vi "Read Result Data.vi"(8 "Error In":errorcluster, 10 "Modbus ID":string, 11 "VISA resource name":refnum<visa-resource-name>) -> (0 "Error Out":errorcluster, 2 "AFV-P Result Data":T1 {"PF" format="%.3f"; "CF" format="%.2f"; "AP" format="%.1f A"; "Q" format="%.1f VAR"; "VA" format="%.1f VA"; "P" format="%.1f W"; "A" format="%.3f A"; "Voltage" format="%.1f V"; "Frequency" format="%.1f Hz"; "Time" format="%.1f s"}, 3 "VISA resource name out":refnum<visa-resource-name>)   [LabVIEW 2013]
panel:
  out "cr_dot":enum16{"CURR_XX_XX", "CURR_X_XXX"}(ring)
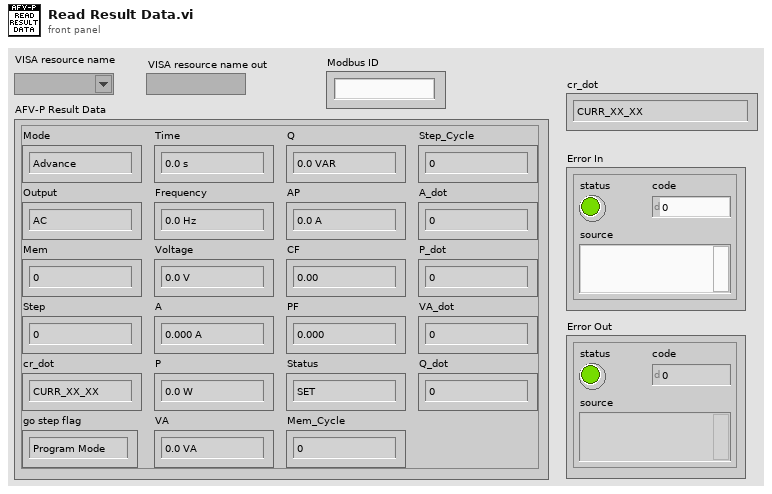
[diagram p1: front panel]
types:
  T1 = cluster{"Mode":enum16{"Advance", "Basic"}, "Output":enum16{"AC", "DC"}, "Mem":u8, "Step":u8, "go step flag":enum16{"Program Mode", "Ganaral Mode"}, "cr_dot":enum16{"CURR_XX_XX", "CURR_X_XXX"}, "Time":dbl, "Frequency":dbl, "Voltage":dbl, "A":dbl, "P":dbl, "VA":dbl, "Q":dbl, "AP":dbl, "CF":dbl, "PF":dbl, "Status":enum16{"SET", "RUNNING", "TRANSIENT", "RAMP", "DELAY", "DWELL", "PASS", "ABORT", "OCP", "A HI LIMIT", "A LO LIMIT", "VA HI LIMIT", "VA LO LIMIT", "AP HI LIMIT", "AP LO LIMIT", "P HI LIMIT", "P LO LIMIT", "PF HI LIMIT", "PF LO LIMIT", "Q HI LIMIT", "Q LO LIMIT", "CF HI LIMIT", "CF LO LIMIT", "AMP STD", "FAN FAIL", "HW OVP", "OVP", "LVP", "FA HI", "FAIL", "OPP", "FREQ-FAIL"}, "Mem_Cycle":u16, "Step_Cycle":u16, "A_dot":u8, "P_dot":u8, "VA_dot":u8, "Q_dot":u8}
  T2 = cluster{"ID":string, "Function Code":string, "Length (High)":string, "Length (Low)":string, "Start Address (High)":string, "Start Address (Middle High)":string, "Start Address (Middle Low)":string, "Start Address (Low)":string, "Data":string}
  T3 = cluster{"Length (High)":string, "Length (Low)":string, "Start Address (High)":string, "Start Address (Middle High)":string, "Start Address (Middle Low)":string, "Start Address (Low)":string}
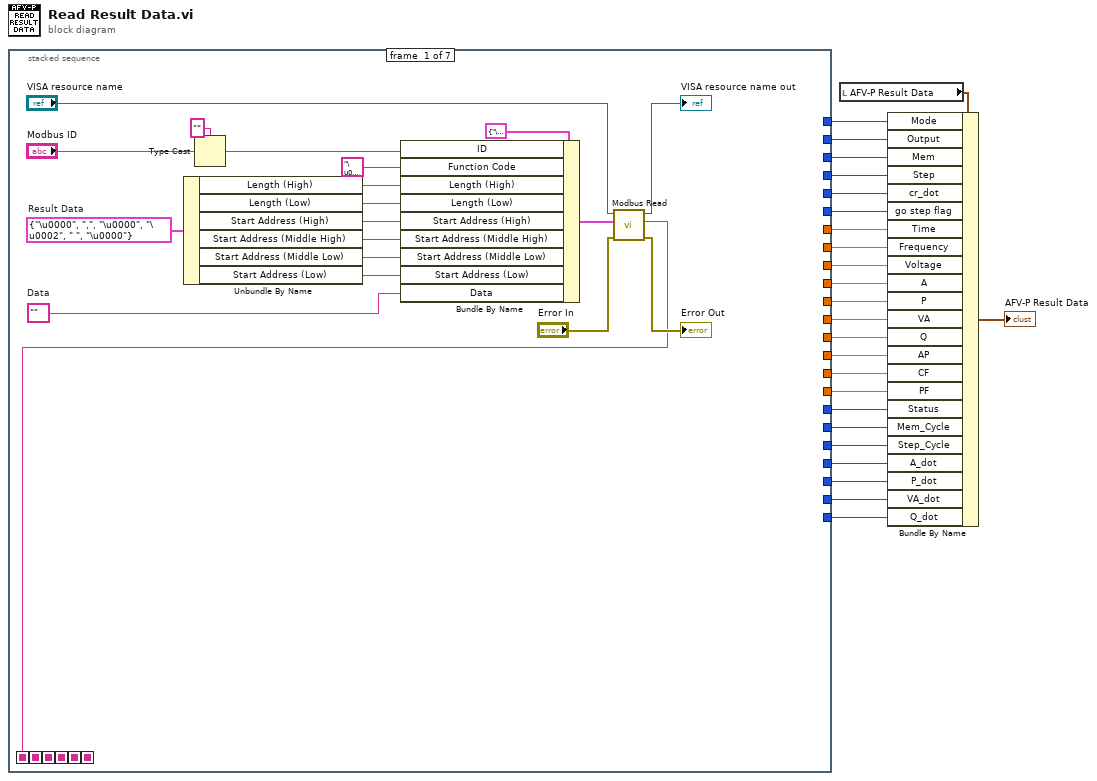
[diagram p0: block diagram]
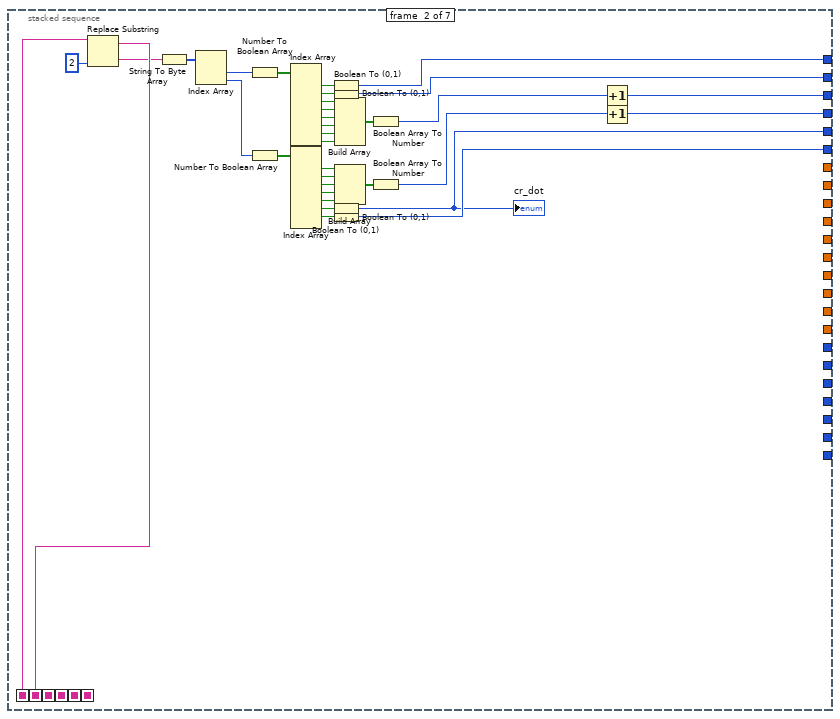
[diagram p2: hidden frame]
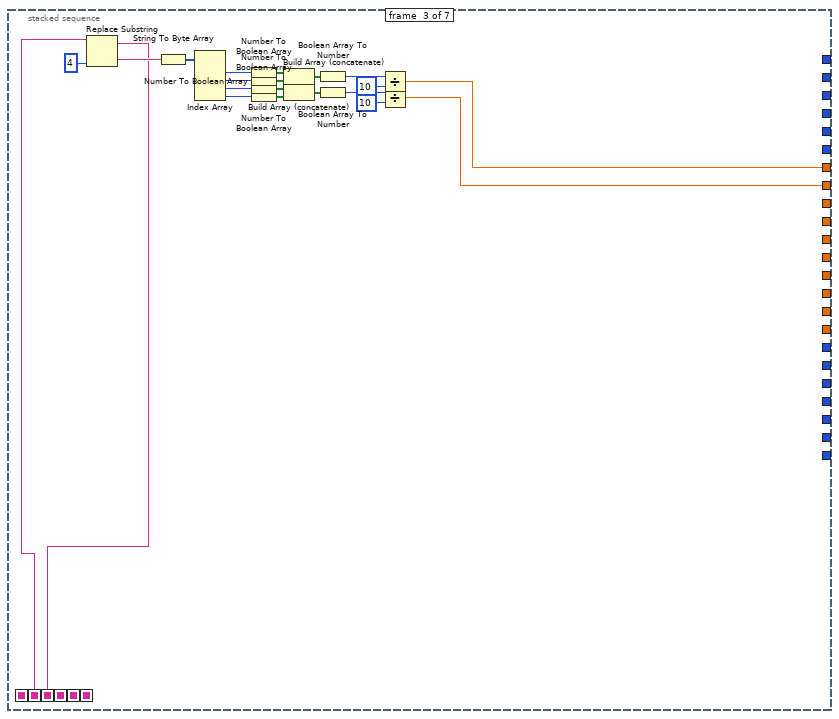
[diagram p3: hidden frame]
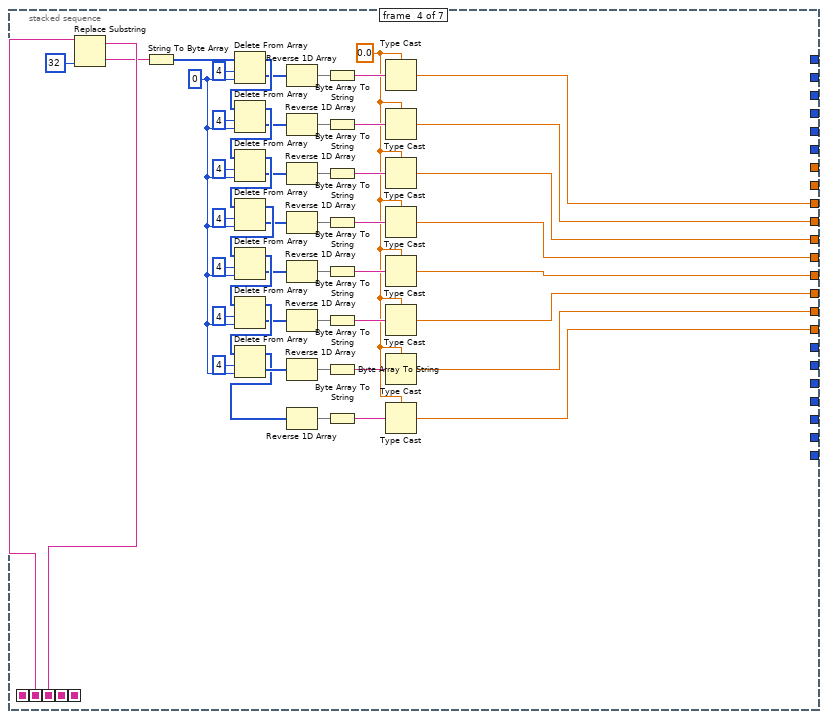
[diagram p4: hidden frame]
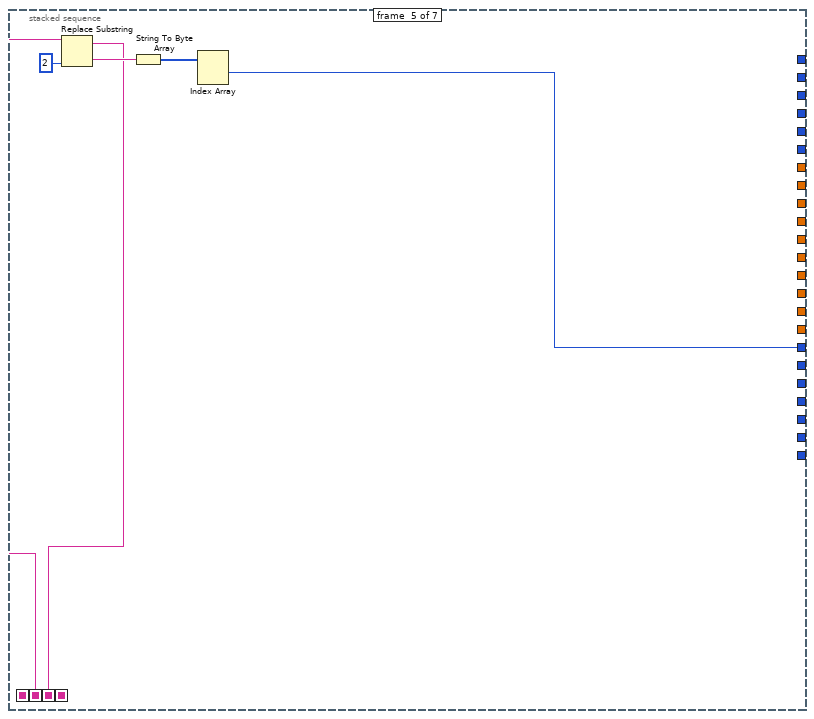
[diagram p5: hidden frame]
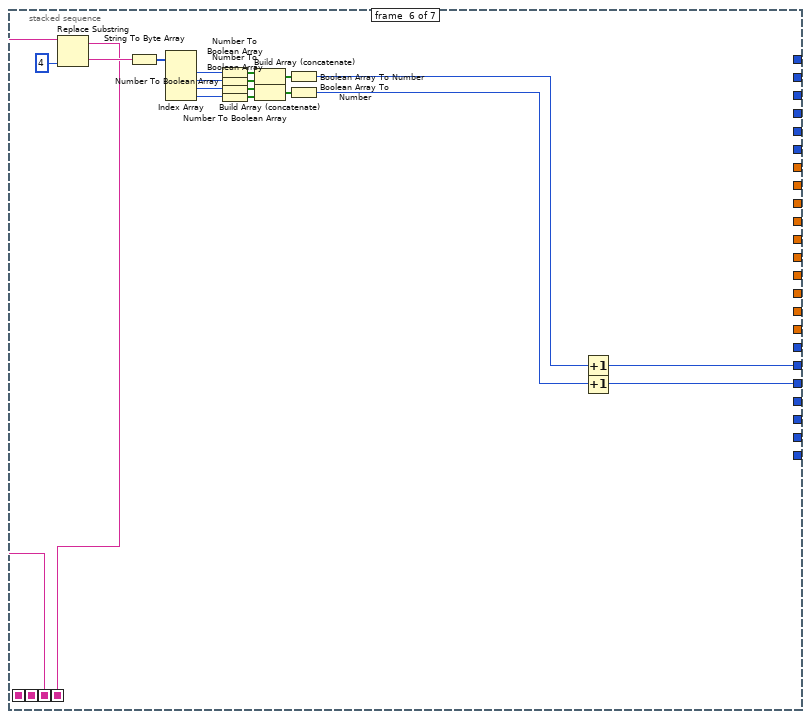
[diagram p6: hidden frame]
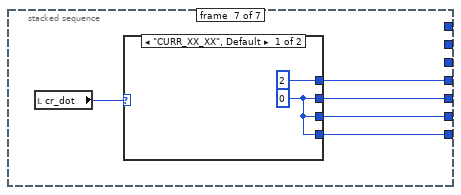
[diagram p7: hidden frame]
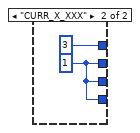
[diagram p8: hidden frame]
diagram:
  n1 = stacked-sequence {
    seq-local: [w32 _ _ _ _ _ _] -> [_ w77 _ _ _ _ _]
    seq-local: [_ w76 _ _ _ _ _] -> [_ _ w95 _ _ _ _]
    seq-local: [_ _ w96 _ _ _ _] -> [_ _ _ w149 _ _ _]
    seq-local: [_ _ _ w150 _ _ _] -> [_ _ _ _ w154 _ _]
    seq-local: [_ _ _ _ w155 _ _] -> [_ _ _ _ _ w173 _]
    seq-local: [_ _ _ _ _ w174 _] -> [_ _ _ _ _ _ _]
    tunnel: [_ w65 _ _ _ _ _] -> w25
    tunnel: [_ w49 _ _ _ _ _] -> w24
    tunnel: [_ w48 _ _ _ _ _] -> w23
    tunnel: [_ w45 _ _ _ _ _] -> w22
    tunnel: [_ _ w87 _ _ _ _] -> w21
    tunnel: [_ _ w79 _ _ _ _] -> w20
    tunnel: [_ w66 _ _ _ _ _] -> w19
    tunnel: [_ _ _ w146 _ _ _] -> w18
    tunnel: [_ _ _ w109 _ _ _] -> w17
    tunnel: [_ _ _ w108 _ _ _] -> w16
    tunnel: [_ _ _ w107 _ _ _] -> w15
    tunnel: [_ _ _ w106 _ _ _] -> w14
    tunnel: [_ _ _ w105 _ _ _] -> w13
    tunnel: [_ _ _ w104 _ _ _] -> w12
    tunnel: [_ _ _ w103 _ _ _] -> w11
    tunnel: [_ _ _ _ w152 _ _] -> w3
    tunnel: [_ _ _ _ _ w159 _] -> w10
    tunnel: [_ _ _ _ _ w158 _] -> w9
    tunnel: [_ _ _ _ _ _ w181] -> w8
    tunnel: [_ _ _ _ _ _ w180] -> w7
    tunnel: [_ _ _ _ _ _ w179] -> w6
    tunnel: [_ _ _ _ _ _ w178] -> w5
    tunnel: [_ w46 _ _ _ _ _] -> w4
    frame #0 {
      w26 = T3 {"Length (High)"="\u0000", "Length (Low)"=",", "Start Address (High)"="\u0000", "Start Address (Middle High)"="\u0002", "Start Address (Middle Low)"=" ", "Start Address (Low)"="\u0000"}  # Result Data
      w43 = ""  # Data
      n2 = Unbundle By Name(w26) -> ("Length (High)"=w42:string, "Length (Low)"=w41:string, "Start Address (High)"=w40:string, "Start Address (Middle High)"=w39:string, "Start Address (Middle Low)"=w38:string, "Start Address (Low)"=w37:string)
      n3 = Type Cast(type="" ("Binary Data (Hex) 3"), x="Modbus ID") -> (*(type *) &x=w28:string)
      n4 = Bundle By Name(cluster=T2 {"ID"="\u0000", "Function Code"="\u0000", "Length (High)"="\u0000", "Length (Low)"="\u0000", "Start Address (High)"="\u0000", "Start Address (Middle High)"="\u0000", "Start Address (Middle Low)"="\u0000", "Start Address (Low)"="\u0000", "Data"=""} ("Write Buffer"), "ID"=w28, "Function Code"="\u0003", "Length (High)"=w42, "Length (Low)"=w41, "Start Address (High)"=w40, "Start Address (Middle High)"=w39, "Start Address (Middle Low)"=w38, "Start Address (Low)"=w37, "Data"=w43) -> (w36:T2)
      n5 = call "Modbus Read.vi"("Error In"="Error In", "Write Buffer"=w36, "VISA resource name"="VISA resource name") -> ("Error Out"=→"Error Out":errorcluster, "Read Data"=w32:string, "VISA resource name out"=→"VISA resource name out":refnum<visa-resource-name>)  [unwired: 6 in]
    }
    frame #1 {
      n6 = Replace Substring(2:2 ("length (len. of substring)"), 5:w77) -> (0:w67:string, 1:w76:string)  [unwired: 2 in]
      n7 = String To Byte Array(string=w67) -> (unsigned byte array=w75:u8[])
      n8 = Index Array(array=w75) -> (element #1=w74:u8, element #2=w52:u8)  [unwired: 2 in]
      n9 = Number To Boolean Array(number=w74) -> (Boolean array=w73:bool[])
      n10 = Number To Boolean Array(number=w52) -> (Boolean array=w53:bool[])
      n11 = Index Array(array=w73) -> (element #1=w72:bool, element #2=w71:bool, element #3=w64:bool, element #4=w63:bool, element #5=w62:bool, element #6=w70:bool, element #7=w69:bool, element #8=w61:bool)  [unwired: 8 in]
      n12 = Index Array(array=w53) -> (element #1=w57:bool, element #2=w58:bool, element #3=w59:bool, element #4=w54:bool, element #5=w55:bool, element #6=w51:bool, element #7=w47:bool)  [unwired: 8 in, 1 out]
      n13 = Boolean To (0,1)(Boolean=w72) -> (0, 1=w66:i16)
      n14 = Boolean To (0,1)(Boolean=w71) -> (0, 1=w65:i16)
      n15 = Boolean To (0,1)(Boolean=w51) -> (0, 1=w45:i16)
      "cr_dot" <- w45
      n16 = Boolean To (0,1)(Boolean=w47) -> (0, 1=w46:i16)
      n17 = Build Array(w64, w63, w62, w70, w69, w61) -> (w68:bool[])
      n18 = Build Array(w57, w58, w59, w54, w55) -> (w56:bool[])
      n19 = Boolean Array To Number(Boolean array=w68) -> (number=w60:u32)
      n20 = Boolean Array To Number(Boolean array=w56) -> (number=w50:u32)
      n21 = Increment(x=w60) -> (x+1=w49:u32)
      n22 = Increment(x=w50) -> (x+1=w48:u32)
    }
    frame #2 {
      n23 = Replace Substring(2:4 ("length (len. of substring)"), 5:w95) -> (0:w97:string, 1:w96:string)  [unwired: 2 in]
      n24 = String To Byte Array(string=w97) -> (unsigned byte array=w98:u8[])
      n25 = Index Array(array=w98) -> (element #1=w91:u8, element #2=w90:u8, element #3=w81:u8, element #4=w80:u8)  [unwired: 4 in]
      n26 = Number To Boolean Array(number=w91) -> (Boolean array=w93:bool[])
      n27 = Number To Boolean Array(number=w90) -> (Boolean array=w92:bool[])
      n28 = Number To Boolean Array(number=w81) -> (Boolean array=w83:bool[])
      n29 = Number To Boolean Array(number=w80) -> (Boolean array=w84:bool[])
      n30 = Build Array (concatenate)(w93, w92) -> (w94:bool[])
      n31 = Build Array (concatenate)(w83, w84) -> (w82:bool[])
      n32 = Boolean Array To Number(Boolean array=w94) -> (number=w89:u32)
      n33 = Boolean Array To Number(Boolean array=w82) -> (number=w85:u32)
      n34 = Divide(x=w89, y=u32 10) -> (x/y=w87:dbl)
      n35 = Divide(x=w85, y=u32 10) -> (x/y=w79:dbl)
    }
    frame #3 {
      w100 = 0 ("index")
      w110 = sgl 0.0
      n36 = Replace Substring(2:32 ("length (len. of substring)"), 5:w149) -> (0:w102:string, 1:w150:string)  [unwired: 2 in]
      n37 = String To Byte Array(string=w102) -> (unsigned byte array=w101:u8[])
      n38 = Delete From Array(array=w101, length=4, index=w100) -> (deleted portion=w132:u8[], array with subset deleted=w145:u8[])
      n39 = Delete From Array(array=w145, length=4, index=w100) -> (deleted portion=w117:u8[], array with subset deleted=w139:u8[])
      n40 = Delete From Array(array=w139, length=4, index=w100) -> (deleted portion=w116:u8[], array with subset deleted=w142:u8[])
      n41 = Delete From Array(array=w142, length=4, index=w100) -> (deleted portion=w115:u8[], array with subset deleted=w133:u8[])
      n42 = Delete From Array(array=w133, length=4, index=w100) -> (deleted portion=w114:u8[], array with subset deleted=w134:u8[])
      n43 = Delete From Array(array=w134, length=4, index=w100) -> (deleted portion=w113:u8[], array with subset deleted=w138:u8[])
      n44 = Delete From Array(array=w138, length=4, index=w100) -> (deleted portion=w112:u8[], array with subset deleted=w111:u8[])
      n45 = Reverse 1D Array(array=w132) -> (reversed array=w148:u8[])
      n46 = Reverse 1D Array(array=w117) -> (reversed array=w130:u8[])
      n47 = Reverse 1D Array(array=w116) -> (reversed array=w129:u8[])
      n48 = Reverse 1D Array(array=w115) -> (reversed array=w125:u8[])
      n49 = Reverse 1D Array(array=w114) -> (reversed array=w126:u8[])
      n50 = Reverse 1D Array(array=w113) -> (reversed array=w119:u8[])
      n51 = Reverse 1D Array(array=w112) -> (reversed array=w120:u8[])
      n52 = Reverse 1D Array(array=w111) -> (reversed array=w122:u8[])
      n53 = Byte Array To String(unsigned byte array=w148) -> (string=w147:string)
      n54 = Byte Array To String(unsigned byte array=w130) -> (string=w131:string)
      n55 = Byte Array To String(unsigned byte array=w129) -> (string=w128:string)
      n56 = Byte Array To String(unsigned byte array=w125) -> (string=w124:string)
      n57 = Byte Array To String(unsigned byte array=w126) -> (string=w127:string)
      n58 = Byte Array To String(unsigned byte array=w119) -> (string=w118:string)
      n59 = Byte Array To String(unsigned byte array=w120) -> (string=w121:string)
      n60 = Byte Array To String(unsigned byte array=w122) -> (string=w123:string)
      n61 = Type Cast(type=w110, x=w147) -> (*(type *) &x=w146:sgl)
      n62 = Type Cast(type=w110, x=w131) -> (*(type *) &x=w109:sgl)
      n63 = Type Cast(type=w110, x=w128) -> (*(type *) &x=w108:sgl)
      n64 = Type Cast(type=w110, x=w124) -> (*(type *) &x=w107:sgl)
      n65 = Type Cast(type=w110, x=w127) -> (*(type *) &x=w106:sgl)
      n66 = Type Cast(type=w110, x=w118) -> (*(type *) &x=w105:sgl)
      n67 = Type Cast(type=w110, x=w121) -> (*(type *) &x=w104:sgl)
      n68 = Type Cast(type=w110, x=w123) -> (*(type *) &x=w103:sgl)
    }
    frame #4 {
      n69 = Replace Substring(2:2 ("length (len. of substring)"), 5:w154) -> (0:w156:string, 1:w155:string)  [unwired: 2 in]
      n70 = String To Byte Array(string=w156) -> (unsigned byte array=w153:u8[])
      n71 = Index Array(array=w153) -> (element #1=w152:u8)  [unwired: 2 in, 1 out]
    }
    frame #5 {
      n72 = Replace Substring(2:4 ("length (len. of substring)"), 5:w173) -> (0:w175:string, 1:w174:string)  [unwired: 2 in]
      n73 = String To Byte Array(string=w175) -> (unsigned byte array=w162:u8[])
      n74 = Index Array(array=w162) -> (element #1=w169:u8, element #2=w168:u8, element #3=w164:u8, element #4=w163:u8)  [unwired: 4 in]
      n75 = Number To Boolean Array(number=w169) -> (Boolean array=w171:bool[])
      n76 = Number To Boolean Array(number=w168) -> (Boolean array=w170:bool[])
      n77 = Number To Boolean Array(number=w164) -> (Boolean array=w166:bool[])
      n78 = Number To Boolean Array(number=w163) -> (Boolean array=w167:bool[])
      n79 = Build Array (concatenate)(w171, w170) -> (w172:bool[])
      n80 = Build Array (concatenate)(w166, w167) -> (w165:bool[])
      n81 = Boolean Array To Number(Boolean array=w172) -> (number=w161:u32)
      n82 = Boolean Array To Number(Boolean array=w165) -> (number=w160:u32)
      n83 = Increment(x=w161) -> (x+1=w159:u32)
      n84 = Increment(x=w160) -> (x+1=w158:u32)
    }
    frame #6 {
      n85 = local read "cr_dot"() -> (w177:enum16{"CURR_XX_XX", "CURR_X_XXX"})
      n86 = case shown="\"CURR_XX_XX\", Default" w177 {
        tunnel: [u8 2 ("A_dot") u8 3 ("A_dot")] -> w181
        tunnel: [w182 w184] -> w180
        tunnel: [w182 w184] -> w179
        tunnel: [w182 w184] -> w178
        frame "CURR_XX_XX", Default {
          w182 = u8 0 ("A_dot")
        }
        frame "CURR_X_XXX" {
          w184 = u8 1 ("A_dot")
        }
      }
    }
  }
  n87 = local read "AFV-P Result Data"() -> (w1:T1)
  n88 = Bundle By Name(cluster=w1, "Mode"=w19, "Output"=w25, "Mem"=w24, "Step"=w23, "cr_dot"=w22, "go step flag"=w4, "Time"=w21, "Frequency"=w20, "Voltage"=w18, "A"=w17, "P"=w16, "VA"=w15, "Q"=w14, "AP"=w13, "CF"=w12, "PF"=w11, "Status"=w3, "Mem_Cycle"=w10, "Step_Cycle"=w9, "A_dot"=w8, "P_dot"=w7, "VA_dot"=w6, "Q_dot"=w5) -> (→"AFV-P Result Data":T1)
